vi "compute_slopes_on_image_starter.vi"() -> ()   [LabVIEW 2018]
uses:
  Classes/Image/Image.lvclass
  Classes/HasoSlopes/HasoSlopes.lvclass
  Controls/Point2D.ctl
panel:
  out "Y Slopes":sgl[][](graph)
  in  "Image file name":string="Data\\data_image.himg"
  in  "Haso configuration file name":string="Data\\config_file_haso.dat"
  in  "Output file name":string="Data\\data_phase_computation_example.has"
  out "X Slopes":sgl[][](graph)
  out "error out":errorcluster
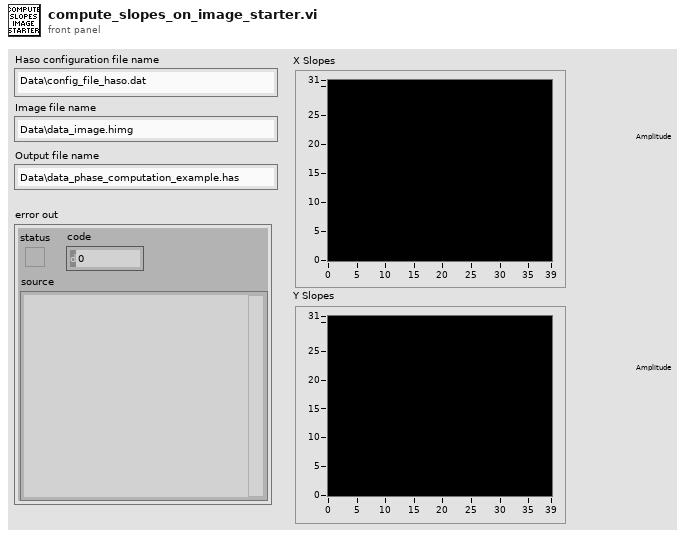
[diagram p1: front panel]
types:
  T1 = typedef "Point2D.ctl" = cluster{"X":u32, "Y":u32}
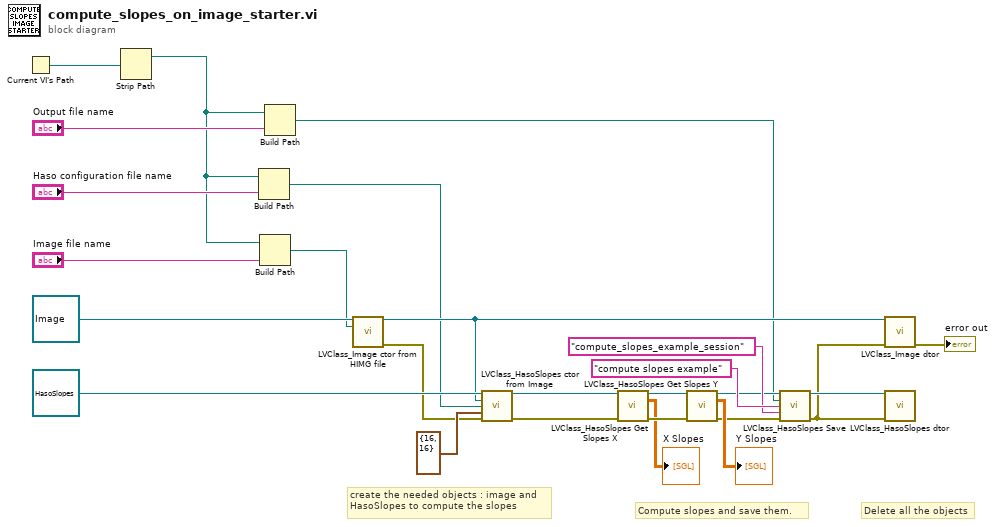
[diagram p0: block diagram]
diagram:
  # "Delete all the objects"
  # "Compute slopes and save them."
  # "create the needed objects : image and\nHasoSlopes to compute the slopes"
  n1 = Current VI's Path() -> (path=w21:path)
  n2 = Strip Path(path=w21) -> (stripped path=w18:path)  [unwired: 1 out]
  n3 = Build Path(base path=w18, name or relative path="Haso configuration file name") -> (appended path=w2:path)
  n4 = Build Path(base path=w18, name or relative path="Image file name") -> (appended path=w1:path)
  n5 = Build Path(base path=w18, name or relative path="Output file name") -> (appended path=w3:path)
  n6 = call "LVClass_Image ctor from HIMG file.vi"("Image (const)"=refnum<class "Image.lvclass"> refnum ("Image in"), "Path to image file"=w1) -> ("Image (new)"=w10:refnum<class "Image.lvclass">, "error out"=w8:errorcluster)  [unwired: 12 in]
  n7 = call "LVClass_HasoSlopes ctor from Image.vi"("HasoSlopes (const)"=refnum<class "HasoSlopes.lvclass"> refnum ("HasoSlopes in"), "Image"=w10, "Haso configuration file"=w2, "start subpupil"=T1 {"X"=16, "Y"=16} ("ImageSize"), "error in (no error)"=w8) -> ("HasoSlopes (new)"=w7:refnum<class "HasoSlopes.lvclass">, "error out"=w4:errorcluster)  [unwired: 8 in, 1 out]
  n8 = call "LVClass_HasoSlopes Get Slopes X.vi"("HasoSlopes in"=w7, "error in (no error)"=w4) -> ("HasoSlopes out"=w17:refnum<class "HasoSlopes.lvclass">, "Slopesx"=→"X Slopes":sgl[][], "error out"=w16:errorcluster)  [unwired: 11 in]
  n9 = call "LVClass_HasoSlopes Get Slopes Y.vi"("HasoSlopes in"=w17, "error in (no error)"=w16) -> ("HasoSlopes out"=w15:refnum<class "HasoSlopes.lvclass">, "Slopesy"=→"Y Slopes":sgl[][], "error out"=w12:errorcluster)  [unwired: 11 in]
  n10 = call "LVClass_HasoSlopes Save.vi"("HasoSlopes in"=w15, "path"=w3, "comments"="compute slopes example", "session"="compute_slopes_example_session", "error in (no error)"=w12) -> ("HasoSlopes out"=w6:refnum<class "HasoSlopes.lvclass">, "error out"=w5:errorcluster)  [unwired: 9 in]
  n11 = call "LVClass_Image dtor.vi"("Image in"=w10, "error in (no error)"=w5) -> ("error out"=→"error out":errorcluster)  [unwired: 12 in, 1 out]
  n12 = call "LVClass_HasoSlopes dtor.vi"("HasoSlopes in"=w6, "error in (no error)"=w5) -> ()  [unwired: 12 in, 2 out]
